vi "TEST6.vi"() -> ()   [LabVIEW 2019]
panel:
  out "Made by":string
  in  "Move/sec":dbl=1.0
  in  "Back":bool
  in  "Forward":bool
  in  "Right":bool
  in  "Left":bool
  in  "Down":bool
  in  "Up":bool
  in  "stop":bool
  out "Data out":string
  in  "TO P0":bool
  in  "P0":string="{0,368,293.5,180,0,90}"
  in  "DO":bool[](array[boolean])
  out "DO number":u32
  out "Data array":string[](array[string])
  in  "Change":bool
  in  "Item":string(combo)
  in  "Value of change":string
  out "Value of Item":string
  out "Data in":string
  out "length":i32
  out "length 2":i32
  out "Data in array":string[](array[string])
  out "index of element":i32
  in  "Port":u16=5000
  in  "Service name":string="192.168.43.45"
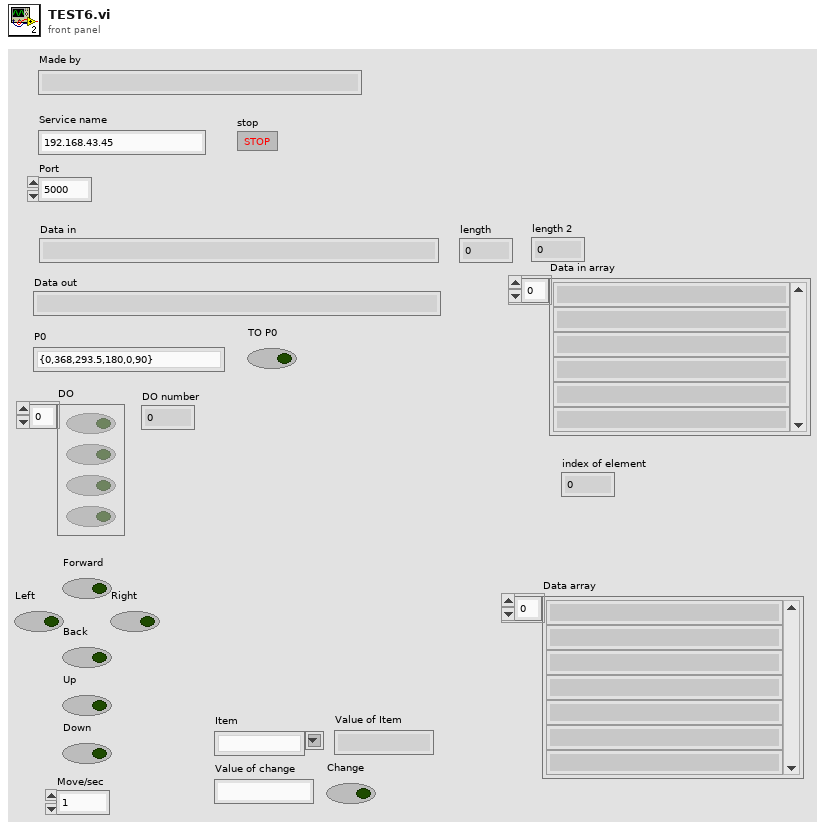
[diagram p1: front panel]
types:
  T1 = enum16{"Standard", "Buffered", "CRLF", "Immediate"}
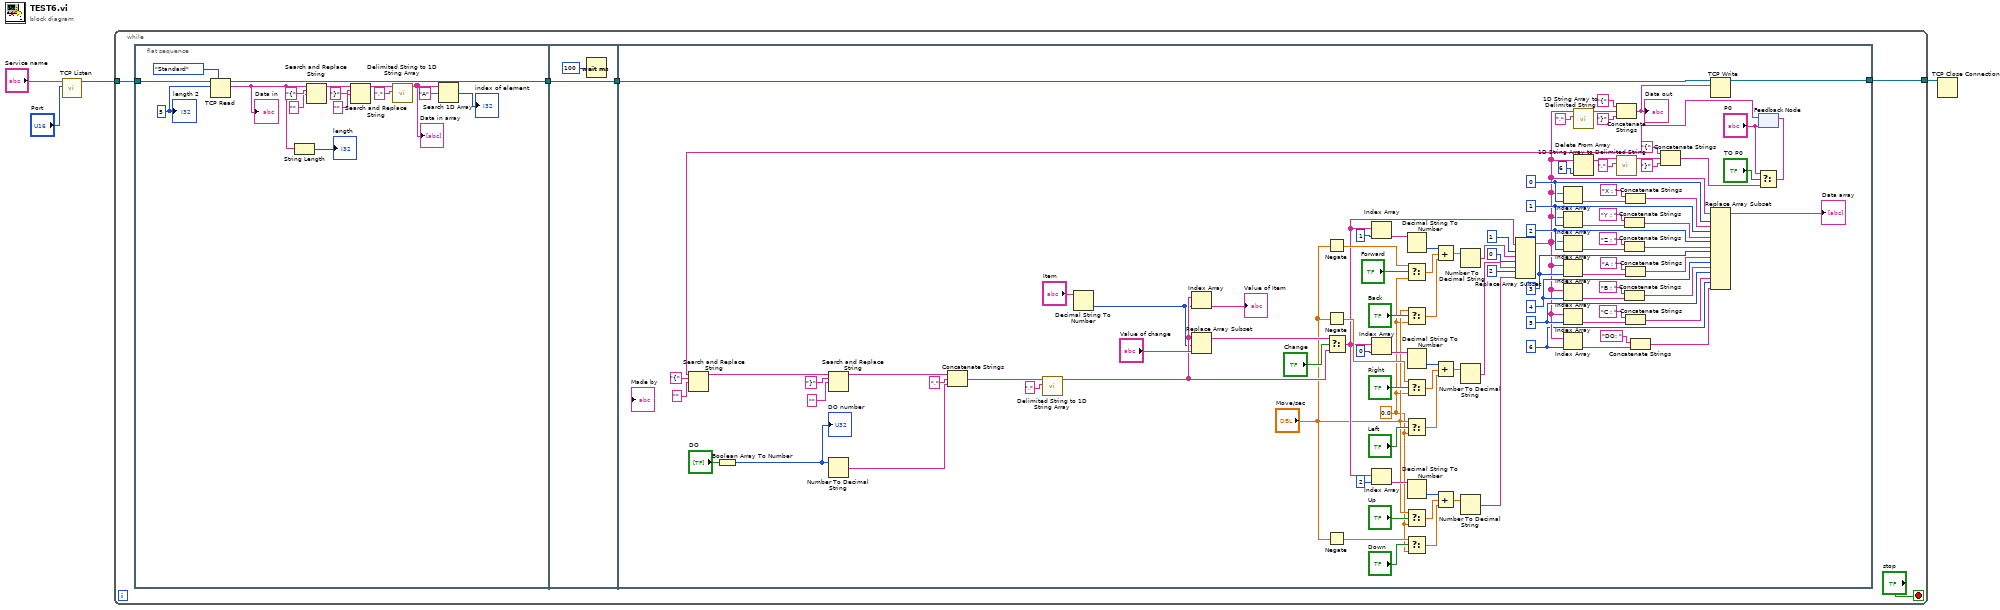
[diagram p0: block diagram]
diagram:
  n1 = call <vilib>:"TCP Listen.vi"("port"="Port", "service name"="Service name") -> ("connection ID"=w1:refnum<k5>)  [unwired: 5 in, 4 out]
  n2 = while {
    tunnel: [w9] -> w2
    tunnel: w1 -> [w5]
    stop <- "stop" stop-if-true
    n3 = flat-sequence {
      tunnel: [w24] -> w6
      tunnel: w5 -> [w25]
      tunnel: [w26] -> w7
      tunnel: w6 -> [w26]
      tunnel: [w130] -> w9
      tunnel: w7 -> [w129]
      frame #0 {
        w22 = 5
        n4 = TCP Read(connection ID=w25, bytes to read=w22, 7:T1."Standard" ("mode (standard)")) -> (connection ID out=w24:refnum<k5>, data out=w13:string)  [unwired: 2 in, 1 out]
        "Data in" <- w13
        n5 = String Length(string=w13) -> (length=→"length":i32)
        n6 = Search and Replace String(input string=w13, search string="{", replace string="" ("replace string (\"\")")) -> (result string=w14:string)  [unwired: 5 in, 3 out]
        n7 = Search and Replace String(input string=w14, search string="}", replace string="" ("replace string (\"\")")) -> (result string=w15:string)  [unwired: 5 in, 3 out]
        n8 = call <vilib>:"Delimited String to 1D String Array.vi"("delimiter"=",", "delimited string"=w15) -> ("string array"=w11:string[])  [unwired: 9 in]
        "Data in array" <- w11
        n9 = Search 1D Array(1D array=w11, element="A") -> (index of element=→"index of element":i32)  [unwired: 1 in]
        "length 2" <- w22
      }
      frame #1 {
        n10 = Wait (ms)(milliseconds to wait=u32 100) -> ()  [unwired: 1 out]
      }
      frame #2 {
        w29 = 6 ("index")
        w34 = 5 ("index")
        w37 = 4 ("index")
        w42 = 3 ("index")
        w45 = 2 ("index")
        w50 = 1 ("index")
        w57 = 0 ("index")
        w64 = 0.0 ("f")
        n11 = Boolean Array To Number(Boolean array="DO") -> (number=w127:u32)
        "DO number" <- w127
        n12 = Number To Decimal String(number=w127) -> (decimal integer string=w105:string)  [unwired: 1 in]
        n13 = Decimal String To Number(string="Item") -> (number=w108:i32)  [unwired: 2 in, 1 out]
        n14 = Negate(x="Move/sec") -> (-x=w83:dbl)
        n15 = Negate(x="Move/sec") -> (-x=w82:dbl)
        n16 = Negate(x="Move/sec") -> (-x=w66:dbl)
        n17 = Select(t=w83, s="Forward", f=w64) -> (s? t:f=w86:dbl)
        n18 = Select(t="Move/sec", s="Back", f=w64) -> (s? t:f=w85:dbl)
        n19 = Select(t=w82, s="Right", f=w64) -> (s? t:f=w77:dbl)
        n20 = Select(t="Move/sec", s="Left", f=w64) -> (s? t:f=w76:dbl)
        n21 = Select(t="Move/sec", s="Up", f=w64) -> (s? t:f=w62:dbl)
        n22 = Select(t=w66, s="Down", f=w64) -> (s? t:f=w61:dbl)
        n23 = feedback #1("P0") -> (w106:string)
        n24 = Search and Replace String(input string=w106, search string="{", replace string="" ("replace string (\"\")")) -> (result string=w121:string)  [unwired: 5 in, 3 out]
        n25 = Search and Replace String(input string=w121, search string="}", replace string="" ("replace string (\"\")")) -> (result string=w107:string)  [unwired: 5 in, 3 out]
        n26 = Concatenate Strings "Concatenate Strings"(w107, "," ("string"), w105) -> (w119:string)
        n27 = call <vilib>:"Delimited String to 1D String Array.vi"("delimiter"=",", "delimited string"=w119) -> ("string array"=w109:string[])  [unwired: 9 in]
        n28 = Index Array "Index Array"(array=w109, index=w108) -> (element=→"Value of Item":string)
        n29 = Replace Array Subset "Replace Array Subset"(array=w109, new element="Value of change", index=w108) -> (w115:string[])
        n30 = Select(t=w115, s="Change", f=w109) -> (s? t:f=w68:string[])
        n31 = Index Array(array=w68, index=1) -> (element=w91:string)
        n32 = Index Array(array=w68, index=0) -> (element=w78:string)
        n33 = Index Array(array=w68, index=2) -> (element=w67:string)
        n34 = Decimal String To Number(string=w91) -> (number=w87:i32)  [unwired: 2 in, 1 out]
        n35 = Decimal String To Number(string=w78) -> (number=w75:i32)  [unwired: 2 in, 1 out]
        n36 = Decimal String To Number(string=w67) -> (number=w63:i32)  [unwired: 2 in, 1 out]
        n37 = Compound Arithmetic op=ADD(w87, w86, w85) -> (w84:dbl)
        n38 = Compound Arithmetic op=ADD(w75, w77, w76) -> (w74:dbl)
        n39 = Compound Arithmetic op=ADD(w63, w62, w61) -> (w60:dbl)
        n40 = Number To Decimal String(number=w84) -> (decimal integer string=w88:string)  [unwired: 1 in]
        n41 = Number To Decimal String(number=w74) -> (decimal integer string=w73:string)  [unwired: 1 in]
        n42 = Number To Decimal String(number=w60) -> (decimal integer string=w59:string)  [unwired: 1 in]
        n43 = Replace Array Subset(array=w68, new element #1=w88, index #1=1 ("index"), new element #2=w73, index #2=0 ("index"), new element #3=w59, index #3=2 ("index")) -> (w30:string[])
        n44 = Index Array(array=w30, index=w57) -> (element=w55:string)
        n45 = Index Array(array=w30, index=w50) -> (element=w51:string)
        n46 = Index Array(array=w30, index=w45) -> (element=w47:string)
        n47 = Index Array(array=w30, index=w42) -> (element=w43:string)
        n48 = Index Array(array=w30, index=w37) -> (element=w39:string)
        n49 = Index Array(array=w30, index=w34) -> (element=w35:string)
        n50 = Index Array(array=w30, index=w29) -> (element=w31:string)
        n51 = call <vilib>:"1D String Array to Delimited String.vi"("delimiter"=",", "string array"=w30) -> ("delimited string"=w112:string)  [unwired: 9 in]
        n52 = Delete From Array(array=w30, index=6) -> (array with subset deleted=w99:string[])  [unwired: 1 in, 1 out]
        n53 = call <vilib>:"1D String Array to Delimited String.vi"("delimiter"=",", "string array"=w99) -> ("delimited string"=w102:string)  [unwired: 9 in]
        n54 = Concatenate Strings("{" ("string"), w112, "}" ("string")) -> (w97:string)
        "Data out" <- w97
        n55 = Concatenate Strings("Y : " ("string"), w51) -> (w49:string)
        n56 = Concatenate Strings("Z : " ("string"), w47) -> (w46:string)
        n57 = Concatenate Strings("B : " ("string"), w39) -> (w38:string)
        n58 = Concatenate Strings("X : " ("string"), w55) -> (w54:string)
        n59 = Concatenate Strings("A : " ("string"), w43) -> (w41:string)
        n60 = Concatenate Strings("C : " ("string"), w35) -> (w33:string)
        n61 = Concatenate Strings("DO: " ("string"), w31) -> (w28:string)
        n62 = Concatenate Strings("{" ("string"), w102, "}" ("string")) -> (w96:string)
        n63 = TCP Write(connection ID=w129, data in=w97) -> (connection ID out=w130:refnum<k5>)  [unwired: 2 in, 2 out]
        n64 = Replace Array Subset "Replace Array Subset"(array=w30, new element #1=w54, index #1=w57, new element #2=w49, index #2=w50, new element #3=w46, index #3=w45, new element #4=w41, index #4=w42, new element #5=w38, index #5=w37, new element #6=w33, index #6=w34, new element #7=w28, index #7=w29) -> (→"Data array":string[])
        n65 = Select(t="P0", s="TO P0", f=w96) -> (s? t:f=w95:string)
        n66 = feedback-in #1(w95) -> ()
      }
    }
  }
  n67 = TCP Close Connection(connection ID=w2) -> ()  [unwired: 2 in, 2 out]
